vi "dcMotor.vi"() -> ()   [LabVIEW 2016]
uses:
  controls/Enum.ctl
  <vilib>/Utility/error.llb/Error Cluster From Error Code.vi
  <vilib>/rvi/errors/niLvFpgaAdjustHostInterfaceError.vi
  <vilib>/rvi/interface/nirviReadWriteControl/nirviReadWriteControl.xnode
  controls/FPGAVIreferenceTypeDef.ctl
  FPGA Bitfiles/qnmController797_usbRIO_controllerFPGAmu.lvbitx
  NiFpgaLv.dll
panel:
  in  "ms":u32=50 format="%.0fms"
  in  "StepMotor":cluster{"Up":bool, "Down":bool}
  in  "DCVoltage":sgl=1.2 format="%#_2pV"
  # "DC Motor"
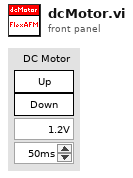
[diagram p1: front panel]
types:
  T1 = typedef "Enum.ctl" = enum16{"Init", "Read", "Write"}
  T2 = typedef "FPGAVIreferenceTypeDef.ctl" = refnum<k20>
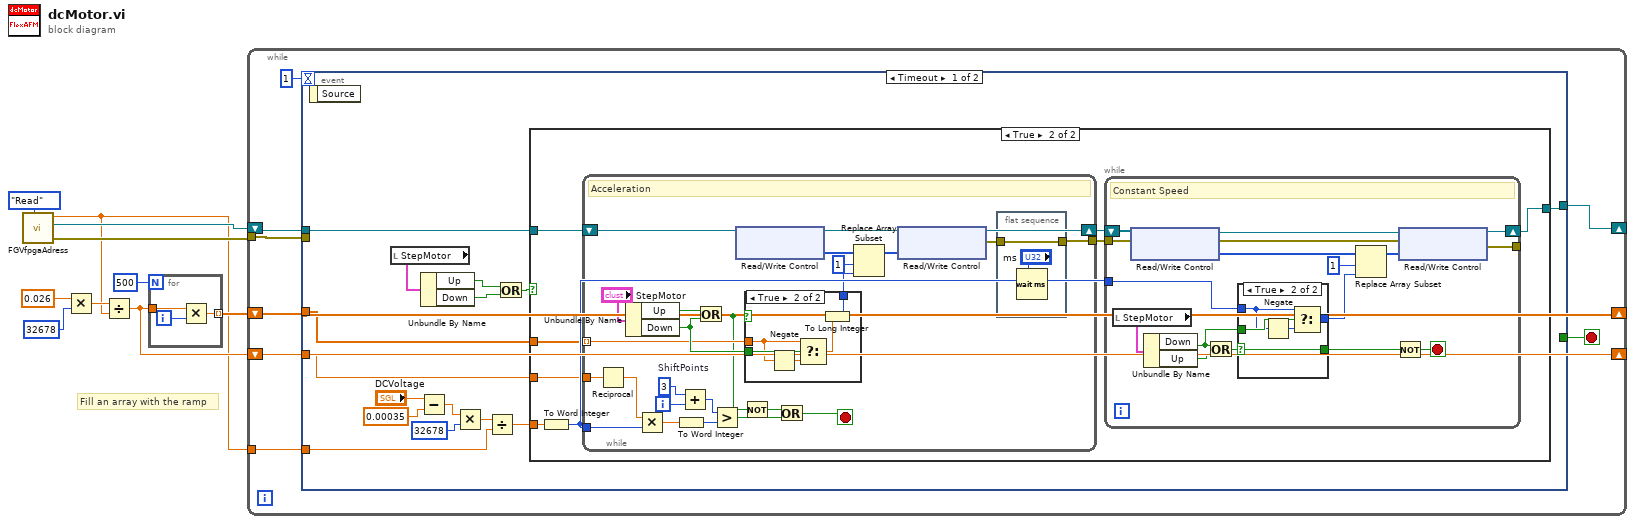
[diagram p0: block diagram]
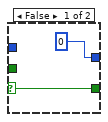
[diagram p3: hidden frame]
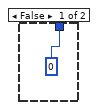
[diagram p4: hidden frame]
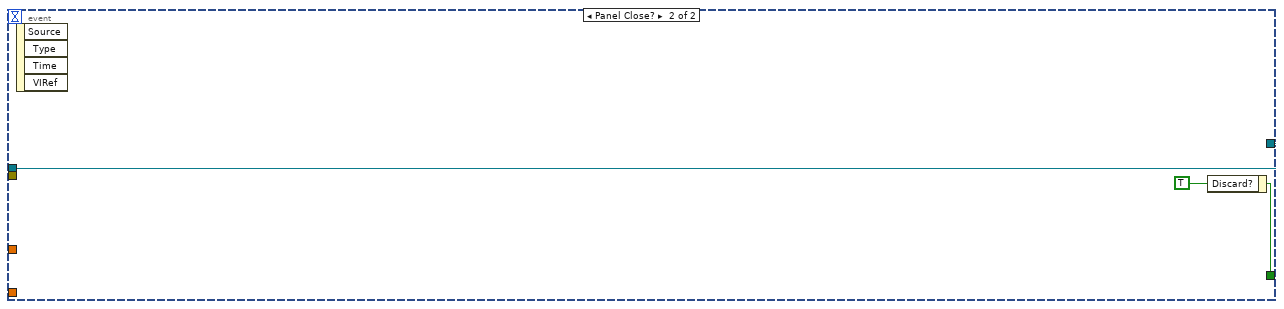
[diagram p5: hidden frame]
diagram:
  # "Fill an array with the ramp"
  n1 = call "FGVfpgaAdress.vi"("Enum"=Enum."Read") -> ("error out"=w8:errorcluster, "FPGA VI Reference Out"=w9:T2, "voltageRange(+/-)Out"=w1:dbl)  [unwired: 5 in, 3 out]
  n2 = Multiply(x=0.026 ("StepSize"), y=32678) -> (x*y=w5:dbl)
  n3 = Divide(x=w5, y=w1) -> (x/y=w2:dbl)
  n4 = for {
    N: 500 -> [_]
    tunnel: w2 -> [w13]
    tunnel: [w11] -> w4 mode=indexing
    i -> [w12]
    n5 = Multiply(x=w13, y=w12) -> (x*y=w11:dbl)
  }
  n6 = while {
    tunnel: w8 -> [w20]
    shift-right: [w18] -> _
    shift-left: w9 -> [w21]
    shift-right: [w17] -> _
    shift-left: w4 -> [w17]
    shift-right: [w16] -> _
    shift-left: w2 -> [w16]
    tunnel: w1 -> [w14]
    stop <- w19 stop-if-true
    n7 = event shown="[0] Timeout" {
      selector: _ -> [_ _]
      dyn-events: _ -> [_ _]
      timeout: 1 -> [_ _]
      tunnel: w17 -> [w28 _]
      tunnel: w21 -> [w29 w103]
      tunnel: w20 -> [_ _]
      tunnel: [_ w104] -> w19
      tunnel: [w30 w103] -> w18
      tunnel: w16 -> [w27 _]
      tunnel: w14 -> [w22 _]
      event Timeout {
        n8 = event-data() -> ()  [unwired: 1 in, 1 out]
        n9 = local read "StepMotor"() -> (w23:cluster{"Up":bool, "Down":bool})
        n10 = Subtract(x="DCVoltage", y=0.00035 ("Offset")) -> (x-y=w36:dbl)
        n11 = Unbundle By Name(w23) -> ("Up"=w26:bool, "Down"=w25:bool)
        n12 = Multiply(x=w36, y=i16 32678) -> (x*y=w32:dbl)
        n13 = Divide(x=w32, y=w22) -> (x/y=w33:dbl)
        n14 = Or(x=w26, y=w25) -> (x .or. y?=w24:bool)
        n15 = case shown="True" w24 {
          tunnel: w33 -> [_ w42]
          tunnel: [w37 w41] -> w30
          tunnel: w29 -> [w37 w40]
          tunnel: w28 -> [_ w39]
          tunnel: w27 -> [_ w38]
          frame False {
          }
          frame True {
            n16 = To Word Integer(number=w42) -> (16bit integer=w45:i16)
            n17 = while {
              tunnel: w39 -> [w86] mode=indexing
              tunnel: [w83] -> w43
              tunnel: w45 -> [w88]
              shift-right: [w84] -> w44
              shift-left: w40 -> [w77]
              tunnel: w38 -> [w80]
              i -> [w94]
              stop <- w70 stop-if-true
              w81 = i16 3  # ShiftPoints
              # "Acceleration"
              n18 = Reciprocal(x=w80) -> (1/x=w93:dbl)
              n19 = Unbundle By Name("StepMotor") -> ("Up"=w92:bool, "Down"=w90:bool)
              n20 = Multiply(x=w93, y=w88) -> (x*y=w87:dbl)
              n21 = To Word Integer(number=w87) -> (16bit integer=w73:i16)
              n22 = Add(x=w81, y=w94) -> (x+y=w82:i32)
              n23 = Or(x=w92, y=w90) -> (x .or. y?=w79:bool)
              n24 = Greater?(x=w82, y=w73) -> (0:w91:bool)
              n25 = xnode "Read/Write Control"("FPGA VI Reference In"=w77) -> ("FPGA VI Reference Out"=w76:T2, "aio.o.outputs"=w75:i16[])  [unwired: 1 in, 1 out]
              n26 = Not(x=w79) -> (.not. x?=w89:bool)
              n27 = case shown="True" w79 {
                tunnel: w90 -> [_ w102]
                tunnel: w86 -> [_ w101]
                tunnel: [0 w98] -> w72
                frame False {
                }
                frame True {
                  n28 = Negate(x=w101) -> (-x=w100:dbl)
                  n29 = Select(t=w101, s=w102, f=w100) -> (s? t:f=w99:dbl)
                  n30 = To Long Integer(number=w99) -> (32bit integer=w98:i32)
                }
              }
              n31 = Or(x=w89, y=w91) -> (x .or. y?=w70:bool)
              n32 = Replace Array Subset(array=w75, new element=w72, index=1) -> (w74:i16[])
              n33 = xnode "Read/Write Control"("FPGA VI Reference In"=w76, "aio.o.outputs"=w74) -> ("FPGA VI Reference Out"=w84:T2, "error out"=w85:errorcluster)  [unwired: 1 in]
              n34 = flat-sequence {
                tunnel: w85 -> [w96]
                tunnel: [w96] -> w83
                frame #0 {
                  n35 = Wait (ms)(milliseconds to wait="ms") -> ()  [unwired: 1 out]
                }
              }
            }
            n36 = while {
              tunnel: w43 -> [w54]
              tunnel: w45 -> [w59]
              shift-right: [w51] -> w41
              shift-left: w44 -> [w55]
              tunnel: [w50] -> _
              stop <- w62 stop-if-true
              # "Constant Speed"
              n37 = local read "StepMotor"() -> (w56:cluster{"Up":bool, "Down":bool})
              n38 = xnode "Read/Write Control"("FPGA VI Reference In"=w55, "error in"=w54) -> ("FPGA VI Reference Out"=w53:T2, "error out"=w52:errorcluster, "aio.o.outputs"=w48:i16[])
              n39 = Unbundle By Name(w56) -> ("Down"=w58:bool, "Up"=w60:bool)
              n40 = Or(x=w58, y=w60) -> (x .or. y?=w61:bool)
              n41 = case shown="True" w61 {
                selector: w61 -> [w63 w65]
                tunnel: w58 -> [_ w69]
                tunnel: w59 -> [_ w68]
                tunnel: [i16 0 w66] -> w47
                tunnel: [w63 w65] -> w57
                frame False {
                }
                frame True {
                  n42 = Negate(x=w68) -> (-x=w67:i16)
                  n43 = Select(t=w68, s=w69, f=w67) -> (s? t:f=w66:i16)
                }
              }
              n44 = Replace Array Subset(array=w48, new element=w47, index=1) -> (w46:i16[])
              n45 = Not(x=w57) -> (.not. x?=w62:bool)
              n46 = xnode "Read/Write Control"("FPGA VI Reference In"=w53, "error in"=w52, "aio.o.outputs"=w46) -> ("FPGA VI Reference Out"=w51:T2, "error out"=w50:errorcluster)
            }
          }
        }
      }
      event Panel Close? {
        w104 = TRUE ("Discard?")
        n47 = event-data() -> ()  [unwired: 1 in, 4 out]
        n48 = event-data("Discard?"=w104) -> ()  [unwired: 1 in, 1 out]
      }
    }
  }
